vi "afmmode.vi"() -> ()   [LabVIEW 2019]
uses:
  <userlib>/HapticSTM/HapticSTM.lvlib
panel:
  out "force":dbl
  out "Z Write (m) 2":dbl
  in  "Z Write?":bool
  in  "Save":bool
  in  "# Sample Points":i32=4096
  out "Signal value":sgl format="%#_6p"
  out "Z Write (m)":dbl
  in  "Signal index (0-127)":i8
  in  "Upper Limit (mm)":dbl=50.0
  in  "Lower Limit (mm)":dbl=-40.0
  in  "Upper Limit (nm)":dbl=1.0
  in  "Lower Limit (nm)":dbl
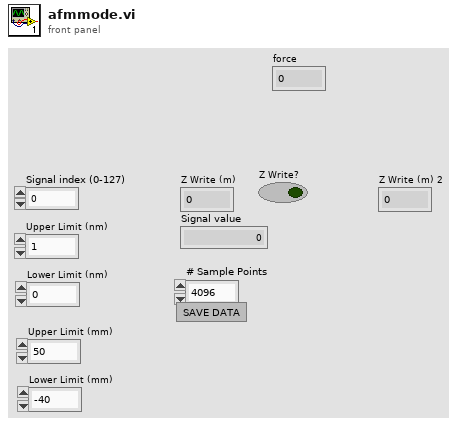
[diagram p1: front panel]
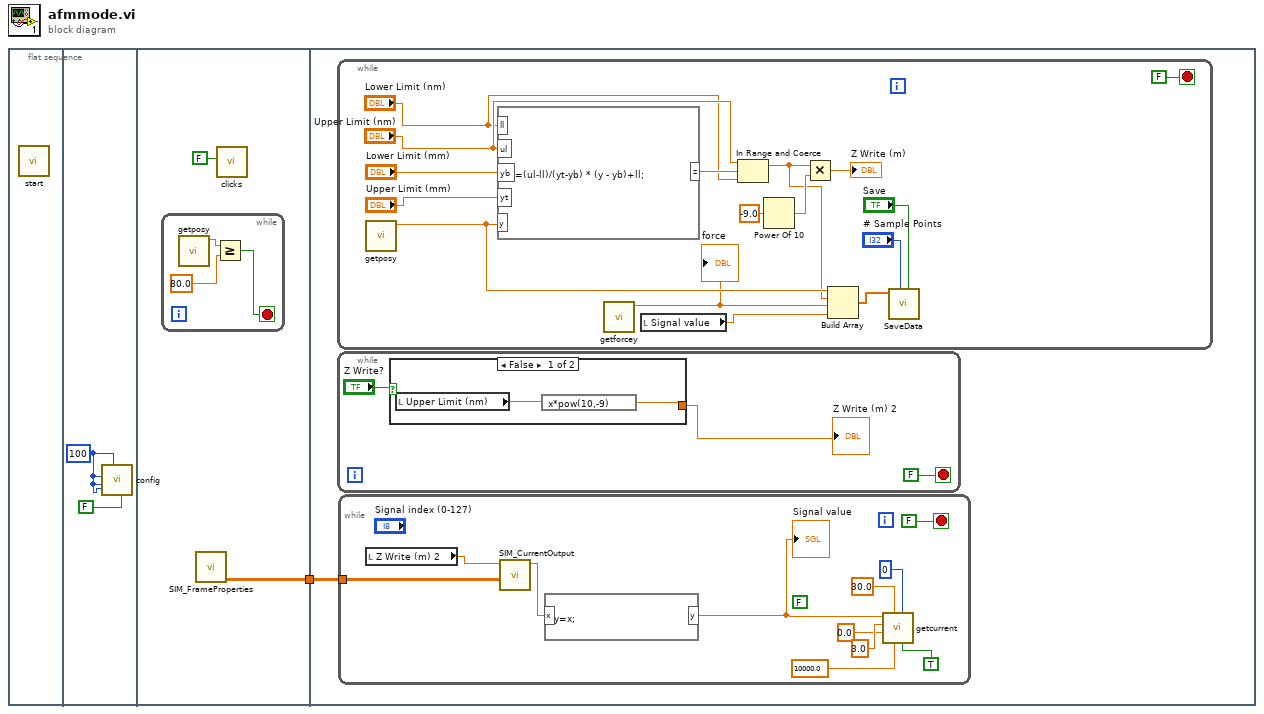
[diagram p0: block diagram]
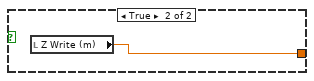
[diagram p2: hidden frame]
diagram:
  n1 = flat-sequence {
    tunnel: [w4] -> w1
    tunnel: w1 -> [w9]
    frame #0 {
      n2 = call <userlib>:"start.vi"() -> ()  [unwired: 11 in, 1 out]
    }
    frame #1 {
      w2 = 100 ("sizeofimgx")
      n3 = call <userlib>:"config.vi"("feedback"=FALSE, "sizeofimgz"=w2, "sizeofimgx"=w2, "scopez"=w2, "scopex"=w2) -> ()  [unwired: 7 in]
    }
    frame #2 {
      n4 = while {
        stop <- w6 stop-if-true
        n5 = call <userlib>:"getposy.vi"() -> ("function return"=w8:dbl)  [unwired: 11 in]
        n6 = Greater Or Equal?(x=w8, y=80.0) -> (x >= y?=w6:bool)
      }
      n7 = call "SIM_FrameProperties.vi"() -> ("data"=w4:dbl[][])  [unwired: 10 in, 1 out]
      n8 = call <userlib>:"clicks.vi"("planing"=FALSE) -> ()  [unwired: 10 in, 1 out]
    }
    frame #3 {
      n9 = while {
        stop <- FALSE stop-if-true
        n10 = call <userlib>:"getposy.vi"() -> ("function return"=w33:dbl)  [unwired: 11 in]
        n11 = formula code="z =(ul-ll)/(yt-yb) * (y - yb)+ll;"("ll"="Lower Limit (nm)", "ul"="Upper Limit (nm)", "yb"="Lower Limit (mm)", "yt"="Upper Limit (mm)", "y"=w33) -> ("z"=w37:dbl)
        n12 = call <userlib>:"getforcey.vi"() -> ("function return"=w31:dbl)  [unwired: 11 in]
        "force" <- w31
        n13 = local read "Signal value"() -> (w28:sgl)
        n14 = In Range and Coerce(upper limit="Upper Limit (nm)", x=w37, lower limit="Lower Limit (nm)") -> (coerced(x)=w32:dbl)  [unwired: 1 out]
        n15 = Power Of 10(x=-9.0) -> (10^x=w38:dbl)
        n16 = Multiply(x=w32, y=w38) -> (x*y=→"Z Write (m)":dbl)
        n17 = Build Array(w33, w32, w31, w28) -> (w27:dbl[])
        n18 = call "SaveData.vi"("Save"="Save", "# Sample Points"="# Sample Points", "Data"=w27) -> ()  [unwired: 9 in]
      }
      n19 = while {
        stop <- FALSE stop-if-true
        n20 = case shown="False" "Z Write?" {
          tunnel: [w13 w15] -> w12
          frame False {
            n21 = local read "Upper Limit (nm)"() -> (w14:dbl)
            n22 = expression code="x*pow(10,-9)"(w14) -> (w13:dbl)
          }
          frame True {
            n23 = local read "Z Write (m)"() -> (w15:dbl)
          }
        }
        "Z Write (m) 2" <- w12
      }
      n24 = while {
        tunnel: w9 -> [w23]
        stop <- FALSE stop-if-true
        (unwired) FALSE ("feedback")
        n25 = local read "Z Write (m) 2"() -> (w17:dbl)
        n26 = call "SIM_CurrentOutput.vi"("array"=w23, "zin (m)"=w17) -> ("Current Out (pA)"=w22:dbl)  [unwired: 8 in, 1 out]
        n27 = formula code="y=x;"("x"=w22) -> ("y"=w16:dbl)
        "Signal value" <- w16
        n28 = call <userlib>:"getcurrent.vi"("afmmode"=TRUE, "forcemode"=0, "maxcurrentin"=10000.0, "setpoint"=30.0, "minforcey"=0.0, "maxforcey"=3.0, "currentin"=w16) -> ()  [unwired: 5 in]
      }
    }
  }
